vi "4_shift_register.vi"() -> ()   [LabVIEW 2017]
panel:
  out "X-3":dbl
  out "X-2":dbl
  out "X-1":dbl
  out "X":dbl
  in  "stop":bool
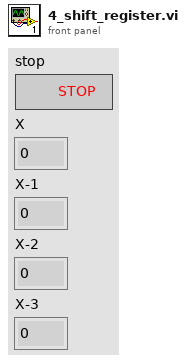
[diagram p1: front panel]
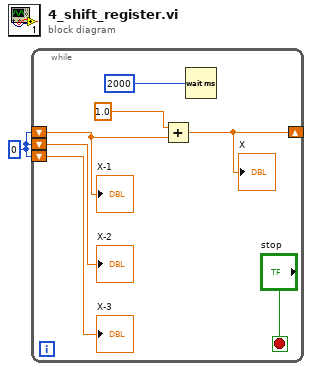
[diagram p0: block diagram]
diagram:
  w1 = 0
  n1 = while {
    shift-right: [w6] -> _
    shift-left: w1 -> [w5]
    shift-left: w1 -> [w3]
    shift-left: w1 -> [w4]
    stop <- "stop" stop-if-true
    n2 = Add(x=1.0, y=w5) -> (x+y=w6:dbl)
    "X" <- w6
    n3 = Wait (ms)(milliseconds to wait=u32 2000) -> ()  [unwired: 1 out]
    "X-1" <- w5
    "X-2" <- w4
    "X-3" <- w3
  }
